vi "Set Cursor Position.vi"(10 "Cursor Position":cluster{"Col":dbl, "Row":dbl}, 11 "Base Graph in":refnum<class "Base Graph.lvclass">) -> (3 "Base Graph out":refnum<class "Base Graph.lvclass">)   [LabVIEW 2023, in "Base Graph.lvclass"]
uses:
  Base Graph.lvclass
  Base Graph.lvclass/Base Graph.ctl
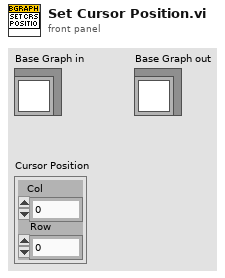
[diagram p1: front panel]
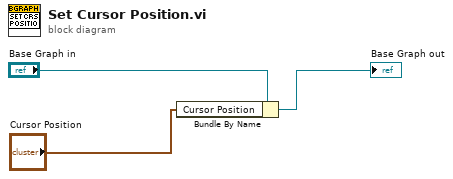
[diagram p0: block diagram]
diagram:
  n1 = Bundle By Name(cluster="Base Graph in", "Cursor Position"="Cursor Position") -> (→"Base Graph out":refnum<class "Base Graph.lvclass">)
